vi "ScriptRequestVI.vi"(4 "Request Name":string, 5 "REPLYTypeDef Path":path, 6 "EventClusterName":string, 7 "REQTypeDef Path":path, 8 "error in (no error)":errorcluster, 10 "Module Ref":refnum<vi>, 11 "VI in":refnum<vi>) -> (0 "error out":errorcluster)   [LabVIEW 2024, in "AddNewEvent.lvlib"]
uses:
  Event/AddNewEvent.lvlib
  <vilib>/Utility/traverseref.llb/TRef TravTarget.ctl
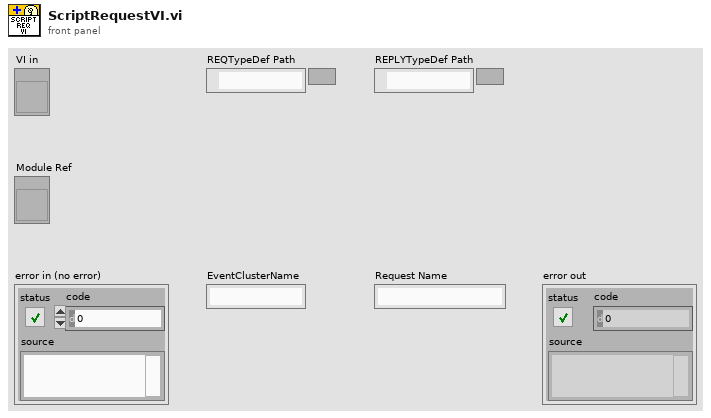
[diagram p1: front panel]
types:
  T1 = typedef "TRef TravTarget.ctl" = enum16{"FP", "BD", "Other"}
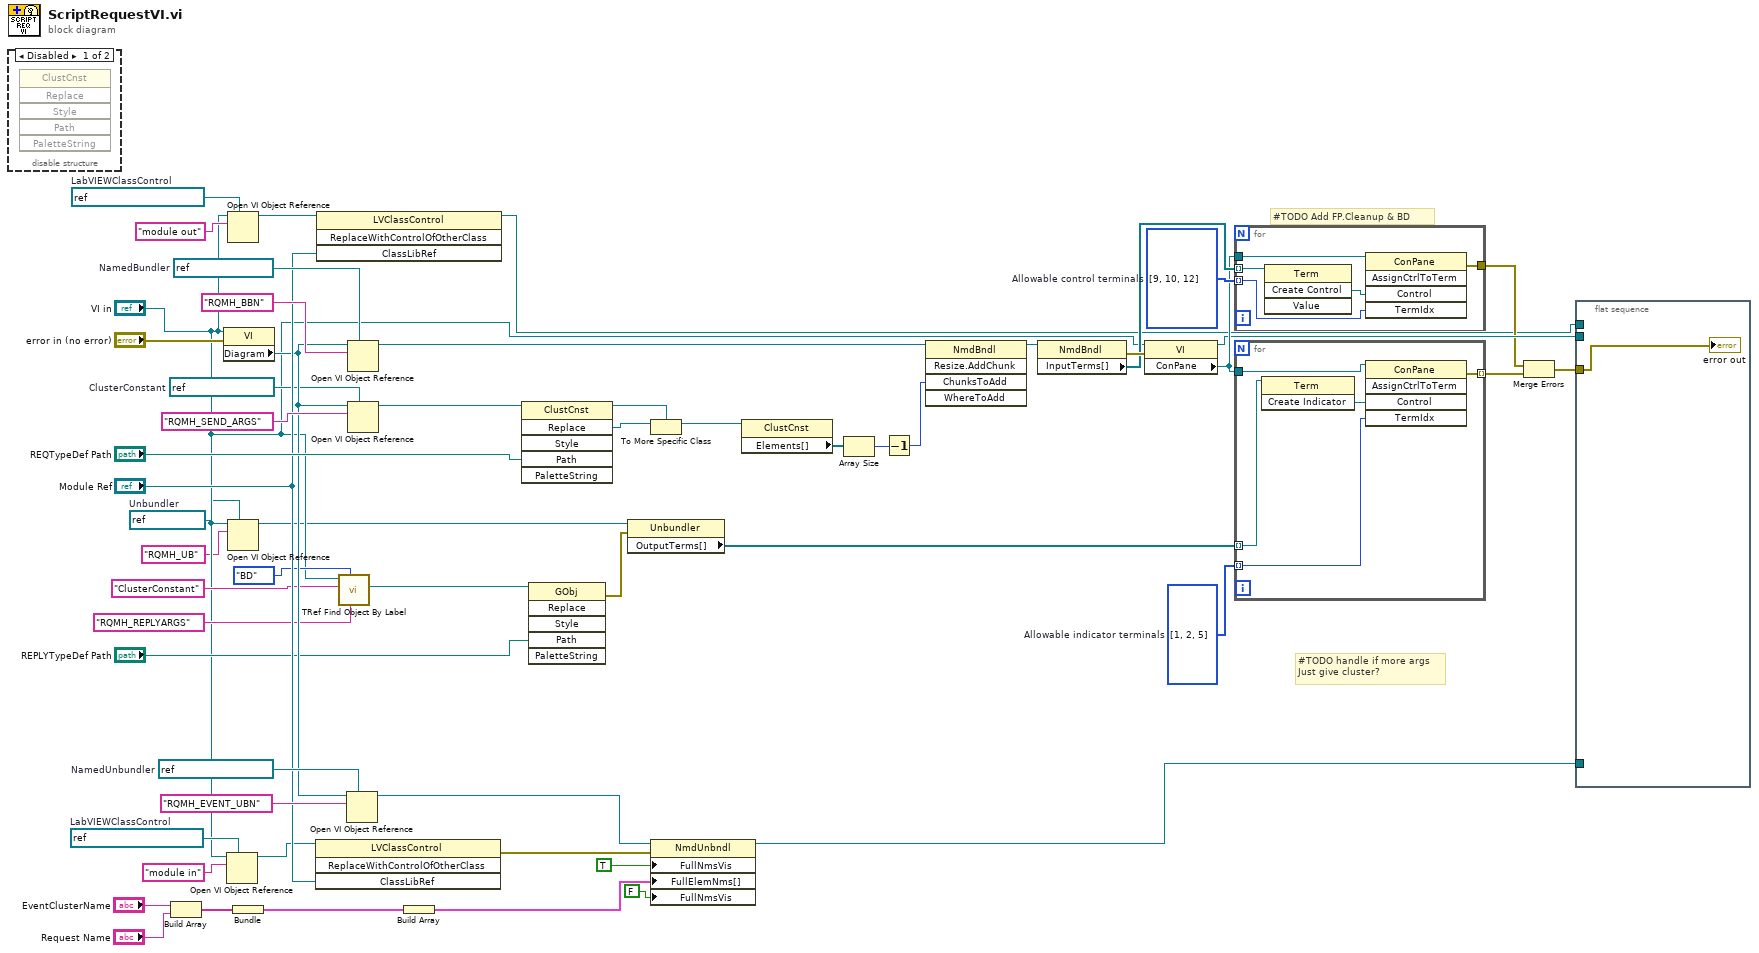
[diagram p0: block diagram]
diagram:
  w11 = i32[] [9, 10, 12]  # Allowable control terminals
  w10 = i32[] [1, 2, 5]  # Allowable indicator terminals
  w14 = refnum<vi> refnum  # Unbundler
  w36 = refnum<vi> refnum  # LabVIEWClassControl
  w33 = refnum<vi> refnum  # LabVIEWClassControl
  w16 = refnum<vi> refnum  # ClusterConstant
  w32 = refnum<vi> refnum  # NamedBundler
  w31 = refnum<vi> refnum  # NamedUnbundler
  # "#TODO handle if more args\nJust give cluster?"
  # "#TODO Add FP.Cleanup & BD"
  n1 = disable-structure shown="Disabled" {
    frame Disabled {
      n2 = invoke class="ClustCnst" method="Replace"() -> ()  [unwired: 6 in, 6 out]
    }
    frame Enabled {
    }
  }
  n3 = Build Array("EventClusterName", "Request Name") -> (w38:string[])
  n4 = property class="VI"(reference="VI in", error in="error in (no error)") -> ("Diagram"=w22:refnum<vi>)  [unwired: 2 out]
  n5 = Open VI Object Reference(7:w33, 10:"module in" ("name/order"), 11:"VI in") -> (3:w23:refnum<vi>)  [unwired: 1 in, 1 out]
  n6 = Open VI Object Reference(7:w36, 10:"module out" ("name/order"), 11:"VI in") -> (3:w37:refnum<vi>)  [unwired: 1 in, 1 out]
  n7 = Open VI Object Reference(7:w14, 10:"RQMH_UB" ("name/order"), 11:"VI in") -> (3:w12:refnum<vi>)  [unwired: 1 in, 1 out]
  n8 = Bundle(w38) -> (w39:cluster{string[]})  [unwired: 1 in]
  n9 = invoke class="LVClassControl" method="ReplaceWithControlOfOtherClass"(reference=w23, "ClassLibRef"="Module Ref") -> (error out=w52:errorcluster)  [unwired: 2 in, 3 out]
  n10 = invoke class="LVClassControl" method="ReplaceWithControlOfOtherClass"(reference=w37, "ClassLibRef"="Module Ref") -> (reference out=w2:refnum<vi>)  [unwired: 2 in, 3 out]
  n11 = call <vilib>:"TRef Find Object By Label.vi"("Label"="RQMH_REPLYARGS" ("name/order"), "Traverse Target"=TRef_TravTarget."BD", "Class Name"="ClusterConstant", "VI Ref"="VI in") -> ("Found Obj Ref"=w18:refnum<vi>)  [unwired: 4 in, 3 out]
  n12 = Open VI Object Reference(7:w31, 10:"RQMH_EVENT_UBN" ("name/order"), 11:w22) -> (3:w40:refnum<vi>)  [unwired: 1 in, 1 out]
  n13 = Open VI Object Reference(7:w32, 10:"RQMH_BBN" ("name/order"), 11:w22) -> (3:w44:refnum<vi>)  [unwired: 1 in, 1 out]
  n14 = Open VI Object Reference(7:w16, 10:"RQMH_SEND_ARGS" ("name/order"), 11:w22) -> (3:w43:refnum<vi>)  [unwired: 1 in, 1 out]
  n15 = Build Array(w39) -> (w41:cluster{string[]}[])
  n16 = invoke class="ClustCnst" method="Replace"(reference=w43, "Path"="REQTypeDef Path") -> (reference out=w49:refnum<vi>, "Replace"=w47:refnum<vi>)  [unwired: 4 in, 4 out]
  n17 = invoke class="GObj" method="Replace"(reference=w18, "Path"="REPLYTypeDef Path") -> (error out=w7:errorcluster)  [unwired: 4 in, 5 out]
  n18 = property class="Unbundler"(reference=w12, error in=w7) -> ("OutputTerms[]"=w9:refnum<vi>[])  [unwired: 2 out]
  n19 = To More Specific Class(target class=w49, reference=w47) -> (specific class reference=w48:refnum<vi>)  [unwired: 1 in, 1 out]
  n20 = property class="NmdUnbndl"(reference=w40, error in=w52, "FullNmsVis"=TRUE ("Full Names Visible?"), "FullElemNms[]"=w41, "FullNmsVis"=FALSE ("Full Names Visible?")) -> (reference out=w1:refnum<vi>)  [unwired: 1 out]
  n21 = property class="ClustCnst"(reference=w48) -> ("Elements[]"=w45:refnum<vi>[])  [unwired: 1 in, 2 out]
  n22 = Array Size(array=w45) -> (size(s)=w46:i32)
  n23 = Decrement(x=w46) -> (x-1=w50:i32)
  n24 = invoke class="NmdBndl" method="Resize.AddChunk"(reference=w44, "ChunksToAdd"=w50) -> (reference out=w51:refnum<vi>)  [unwired: 3 in, 4 out]
  n25 = property class="NmdBndl"(reference=w51) -> (error out=w55:errorcluster, "InputTerms[]"=w25:refnum<vi>[])  [unwired: 1 in, 1 out]
  n26 = property class="VI"(reference="VI in", error in=w55) -> (reference out=w6:refnum<vi>, "ConPane"=w8:refnum<vi>)  [unwired: 1 out]
  n27 = for {
    tunnel: w8 -> [w61]
    tunnel: [w60] -> w5
    tunnel: w25 -> [w59] mode=indexing
    tunnel: w11 -> [w58] mode=indexing
    n28 = invoke class="Term" method="Create Control"(reference=w59) -> ("Create Control"=w57:refnum<vi>)  [unwired: 3 in, 3 out]
    n29 = invoke class="ConPane" method="AssignCtrlToTerm"(reference=w61, "Control"=w57, "TermIdx"=w58) -> (error out=w60:errorcluster)  [unwired: 2 in, 4 out]
  }
  n30 = for {
    tunnel: w8 -> [w66]
    tunnel: w9 -> [w64] mode=indexing
    tunnel: w10 -> [w63] mode=indexing
    tunnel: [w62] -> w4 mode=indexing
    n31 = invoke class="Term" method="Create Indicator"(reference=w64) -> ("Create Indicator"=w65:refnum<vi>)  [unwired: 2 in, 2 out]
    n32 = invoke class="ConPane" method="AssignCtrlToTerm"(reference=w66, "Control"=w65, "TermIdx"=w63) -> (error out=w62:errorcluster)  [unwired: 2 in, 4 out]
  }
  n33 = Merge Errors(w5, w4) -> (w3:errorcluster)
  n34 = flat-sequence {
    tunnel: w6 -> [_]
    tunnel: w3 -> [w67]
    tunnel: w2 -> [_]
    tunnel: w1 -> [_]
    frame #0 {
      "error out" <- w67
    }
  }
